vi "SetHeader_ProxyAuthentication.vi"(8 "error in (no error)":errorcluster, 9 "parameter":string, 10 "scheme":string, 11 "HttpHeaders_Request in":refnum<class "HttpHeaders_Request.lvclass">) -> (0 "error out":errorcluster, 3 "HttpHeaders_Request out":refnum<class "HttpHeaders_Request.lvclass">)   [LabVIEW 2018, in "HttpClient_NET.lvlib" / "HttpHeaders_Request.lvclass"]
uses:
  HttpHeaders_Request.lvclass
  C:/Viviota/Projects/R&D/LabVIEW_HTTP_REST_NET/HTTPHeaders_NET/HttpHeaders_NET.lvclass
  System.Net.Http
  HTTPHeaders_NET/HttpHeaders_NET.lvclass/HttpHeaders_NET.ctl
  Read NET_HttpRequestHeaders.vi
  HTTPHeaders_NET/Accessors/Read NET_HttpHeaders.vi
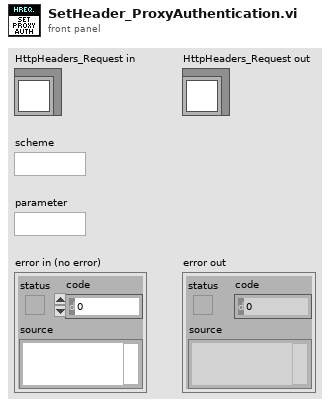
[diagram p1: front panel]
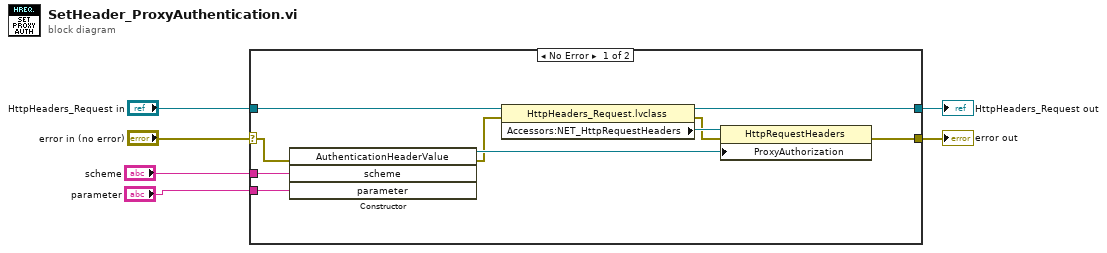
[diagram p0: block diagram]
diagram:
  n1 = case shown="No Error" "error in (no error)" {
    selector: "error in (no error)" -> [w12 w18]
    tunnel: [w7 w18] -> w5
    tunnel: [w15 w17] -> w3
    tunnel: "HttpHeaders_Request in" -> [w16 w17]
    tunnel: "scheme" -> [w9 _]
    tunnel: "parameter" -> [w8 _]
    frame No Error {
      n2 = constructor class="AuthenticationHeaderValue"(error in=w12, "scheme"=w9, "parameter"=w8) -> (reference out=w13:refnum<k24>, error out=w11:errorcluster)  [unwired: 2 in, 3 out]
      n3 = property class="HttpHeaders_Request.lvclass"(reference=w16, error in=w11) -> (reference out=w15:refnum<class "HttpHeaders_Request.lvclass">, error out=w10:errorcluster, "Accessors:NET_HttpRequestHeaders"=w14:refnum<k24>)
      n4 = property class="HttpRequestHeaders"(reference=w14, error in=w10, "ProxyAuthorization"=w13) -> (error out=w7:errorcluster)  [unwired: 1 out]
    }
    frame Error {
    }
  }
  "error out" <- w5
  "HttpHeaders_Request out" <- w3
